vi "Set Visible State on Multiple Controls.vi"(10 "Visble?":bool, 11 "Controls":refnum<vi>[](array[refnum])) -> ()   [LabVIEW 2021]
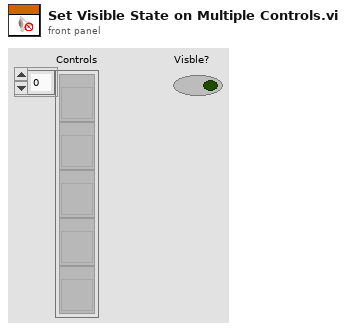
[diagram p1: front panel]
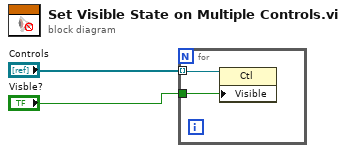
[diagram p0: block diagram]
diagram:
  n1 = for {
    tunnel: "Controls" -> [w4] mode=indexing
    tunnel: "Visble?" -> [w3]
    n2 = property class="Ctl"(reference=w4, "Visible"=w3) -> ()  [unwired: 1 in, 2 out]
  }
